vi "wardsw.vi"(9 "n":i32, 10 "i":i32, 11 "d":dbl[](array[numeric])) -> (3 "d(wardsw)":dbl[](array[numeric]))   [LabVIEW 2014]
panel:
  out "temp":dbl=1.797693134862e+308
  out "k":i32
  out "nn":i32
  out "ii":i32
  out "n1":i32
  out "i1":i32
  out "FLMAX":dbl=1.797693134862e+308
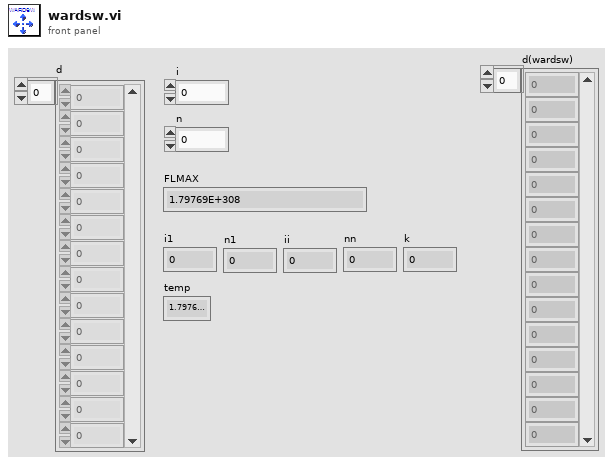
[diagram p1: front panel]
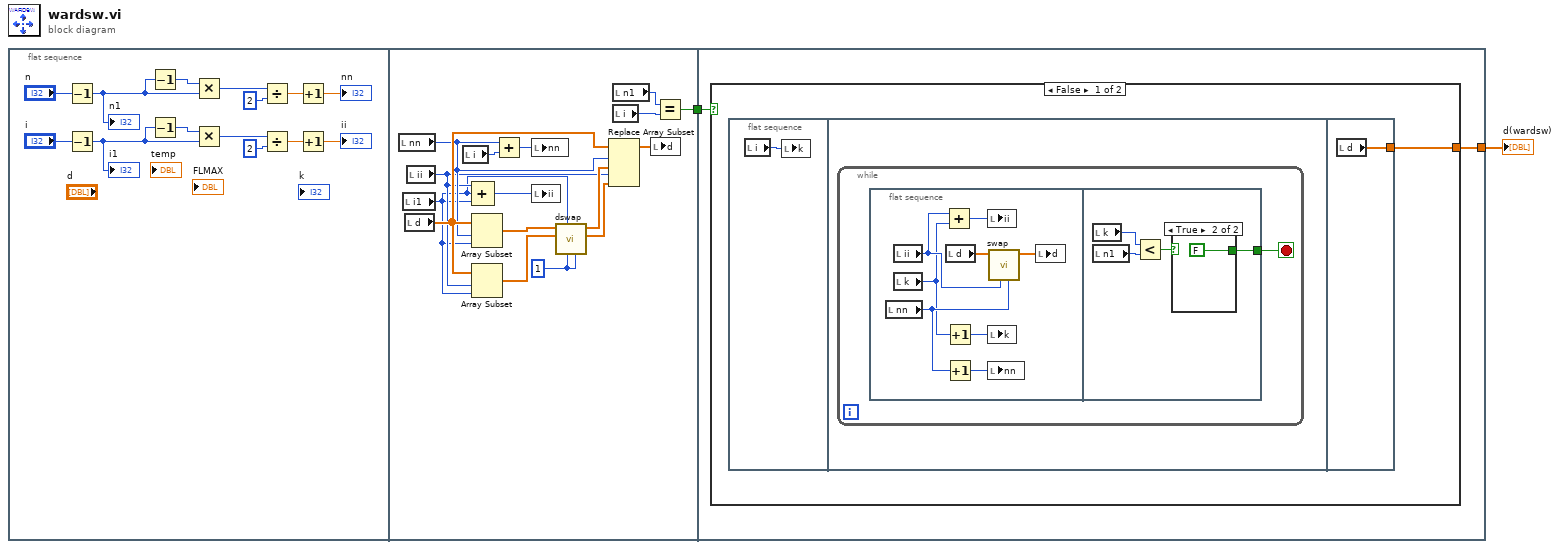
[diagram p0: block diagram]
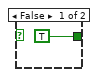
[diagram p2: hidden frame]
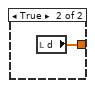
[diagram p3: hidden frame]
diagram:
  n1 = flat-sequence {
    tunnel: [w17] -> w2
    tunnel: w2 -> [w34]
    tunnel: [w33] -> w1
    frame #0 {
      n2 = Decrement(x="n") -> (x-1=w3:i32)
      "n1" <- w3
      n3 = Decrement(x="i") -> (x-1=w14:i32)
      "i1" <- w14
      n4 = Decrement(x=w3) -> (x-1=w6:i32)
      n5 = Decrement(x=w14) -> (x-1=w15:i32)
      n6 = Multiply(x=w6, y=w3) -> (x*y=w7:i32)
      n7 = Multiply(x=w15, y=w14) -> (x*y=w13:i32)
      n8 = Divide(x=w7, y=2) -> (x/y=w9:dbl)
      n9 = Divide(x=w13, y=2) -> (x/y=w11:dbl)
      n10 = Increment(x=w9) -> (x+1=→"nn":dbl)
      n11 = Increment(x=w11) -> (x+1=→"ii":dbl)
    }
    frame #1 {
      w30 = 1 ("incx")
      n12 = local read "nn"() -> (w25:i32)
      n13 = local read "i1"() -> (w21:i32)
      n14 = local read "d"() -> (w27:dbl[])
      n15 = local read "ii"() -> (w22:i32)
      n16 = local read "i"() -> (w24:i32)
      n17 = Compound Arithmetic op=ADD(w22, w21, w21) -> (w20:i32)
      n18 = Array Subset(array=w27, index=w25, length=w21) -> (w32:dbl[])
      n19 = Array Subset(array=w27, index=w22, length=w21) -> (w31:dbl[])
      n20 = Add(x=w25, y=w24) -> (x+y=w23:i32)
      n21 = local write "nn"(w23) -> ()
      n22 = local write "ii"(w20) -> ()
      n23 = call "dswap.vi"("incy"=w30, "incx"=w30, "n"=w21, "dy"=w31, "dx"=w32) -> ("dy_swaped"=w28:dbl[], "dx_swaped"=w29:dbl[])  [unwired: 5 in]
      n24 = Replace Array Subset(array=w27, new element #1=w29, index #1=w25, new element #2=w28, index #2=w22) -> (w26:dbl[])
      n25 = local read "n1"() -> (w18:i32)
      n26 = local read "i"() -> (w19:i32)
      n27 = local write "d"(w26) -> ()
      n28 = Equal?(x=w18, y=w19) -> (x = y?=w17:bool)
    }
    frame #2 {
      n29 = case shown="False" w34 {
        tunnel: [w35 w53] -> w33
        frame False {
          n30 = flat-sequence {
            tunnel: [w52] -> w35
            frame #0 {
              n31 = local read "i"() -> (w36:i32)
              n32 = local write "k"(w36) -> ()
            }
            frame #1 {
              n33 = while {
                stop <- w37 stop-if-true
                n34 = flat-sequence {
                  tunnel: [w49] -> w37
                  frame #0 {
                    n35 = local read "nn"() -> (w43:i32)
                    n36 = local read "ii"() -> (w40:i32)
                    n37 = local read "k"() -> (w39:i32)
                    n38 = Add(x=w40, y=w39) -> (x+y=w38:i32)
                    n39 = Increment(x=w39) -> (x+1=w41:i32)
                    n40 = Increment(x=w43) -> (x+1=w42:i32)
                    n41 = local read "d"() -> (w45:dbl[])
                    n42 = local write "ii"(w38) -> ()
                    n43 = local write "k"(w41) -> ()
                    n44 = local write "nn"(w42) -> ()
                    n45 = call "swap.vi"("j"=w43, "k"=w40, "Array"=w45) -> ("Array (swap)"=w44:dbl[])  [unwired: 8 in]
                    n46 = local write "d"(w44) -> ()
                  }
                  frame #1 {
                    n47 = local read "k"() -> (w48:i32)
                    n48 = local read "n1"() -> (w46:i32)
                    n49 = Less?(x=w48, y=w46) -> (x < y?=w47:bool)
                    n50 = case shown="True" w47 {
                      tunnel: [TRUE FALSE] -> w49
                      frame False {
                      }
                      frame True {
                      }
                    }
                  }
                }
              }
            }
            frame #2 {
              n51 = local read "d"() -> (w52:dbl[])
            }
          }
        }
        frame True {
          n52 = local read "d"() -> (w53:dbl[])
        }
      }
    }
  }
  "d(wardsw)" <- w1
